vi "invatare retea.vi"() -> ()   [LabVIEW 2024]
uses:
  <vilib>/National Instruments/NI Super Simple Neural Networks/Types/Teaching Settings.ctl
  <vilib>/National Instruments/NI Super Simple Neural Networks/Types/Error Evaluation.ctl
  <vilib>/National Instruments/NI Super Simple Neural Networks/API/Create 2 Hidden Layers.vi
  <vilib>/National Instruments/NI Super Simple Neural Networks/Neural Network.lvclass
panel:
  out "F1 SCOR":dbl
  out "Accuracy":dbl
  out "Matrice confuzie":dbl[][](array[numeric])
  in  "Settings In":T1={"Max Epocs"=10000, "Error Goal"=10.0, "Max Time (s)"=10.0, "Error Evaluation"=enum."Over Teaching Set", "# Vectors per Iteration"=200}
  out "Waveform Graph 2":dbl[][](graph)
  out "Solution Found":bool
  out "Error Trend Out":dbl[](array[numeric])
  out "Teaching Time (s)":dbl
  in  "Output Layer Linear (False)":bool
  out "nume clase":string[](array[string])
  in  "2nd Hidden Layer Neurons":u32
  in  "1st Hidden Layer Neurons":u32
  # "250"
  # "60"
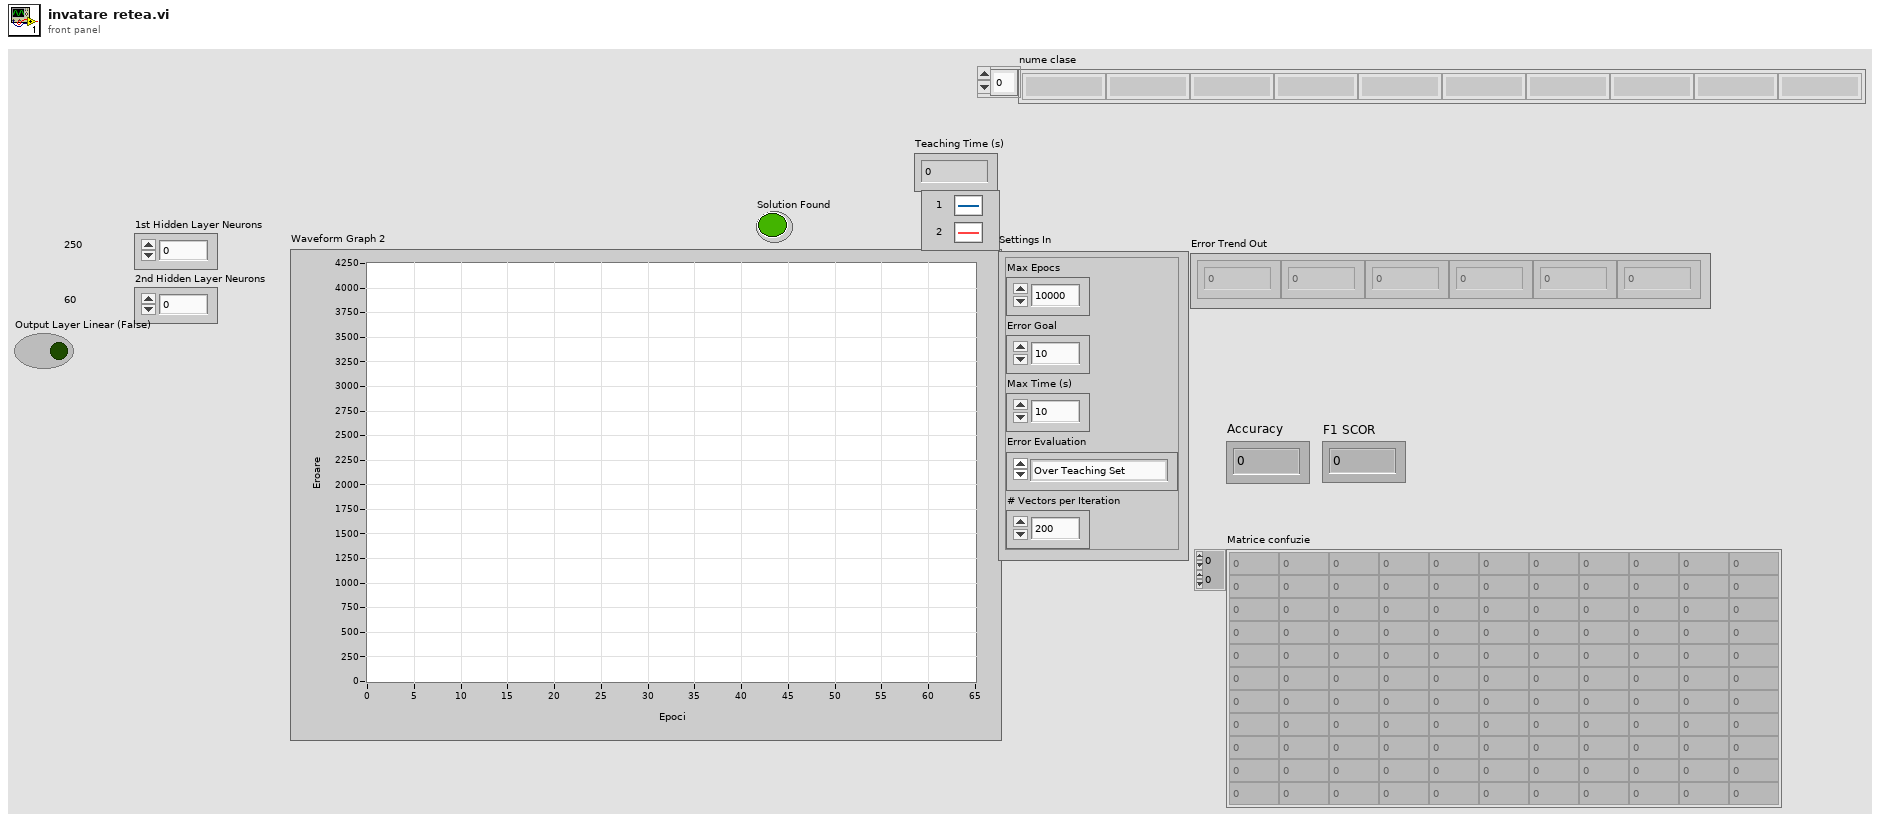
[diagram p1: front panel]
types:
  T1 = typedef "Neural Network.lvclass/Teaching Settings.ctl" = cluster{"Max Epocs":u64, "Error Goal":dbl, "Max Time (s)":dbl, "Error Evaluation":T2, "# Vectors per Iteration":i32}
  T2 = typedef "Neural Network.lvclass/Error Evaluation.ctl" = enum16{"Over Both Sets", "Over Validation Set", "Over Teaching Set"}
  T3 = typedef "imagedata.ctl" = cluster{"image type":i32, "image depth":i32, "image":u8[], "mask":u8[], "colors":u32[], "Rectangle":cluster{"left":i16, "top":i16, "right":i16, "bottom":i16}}
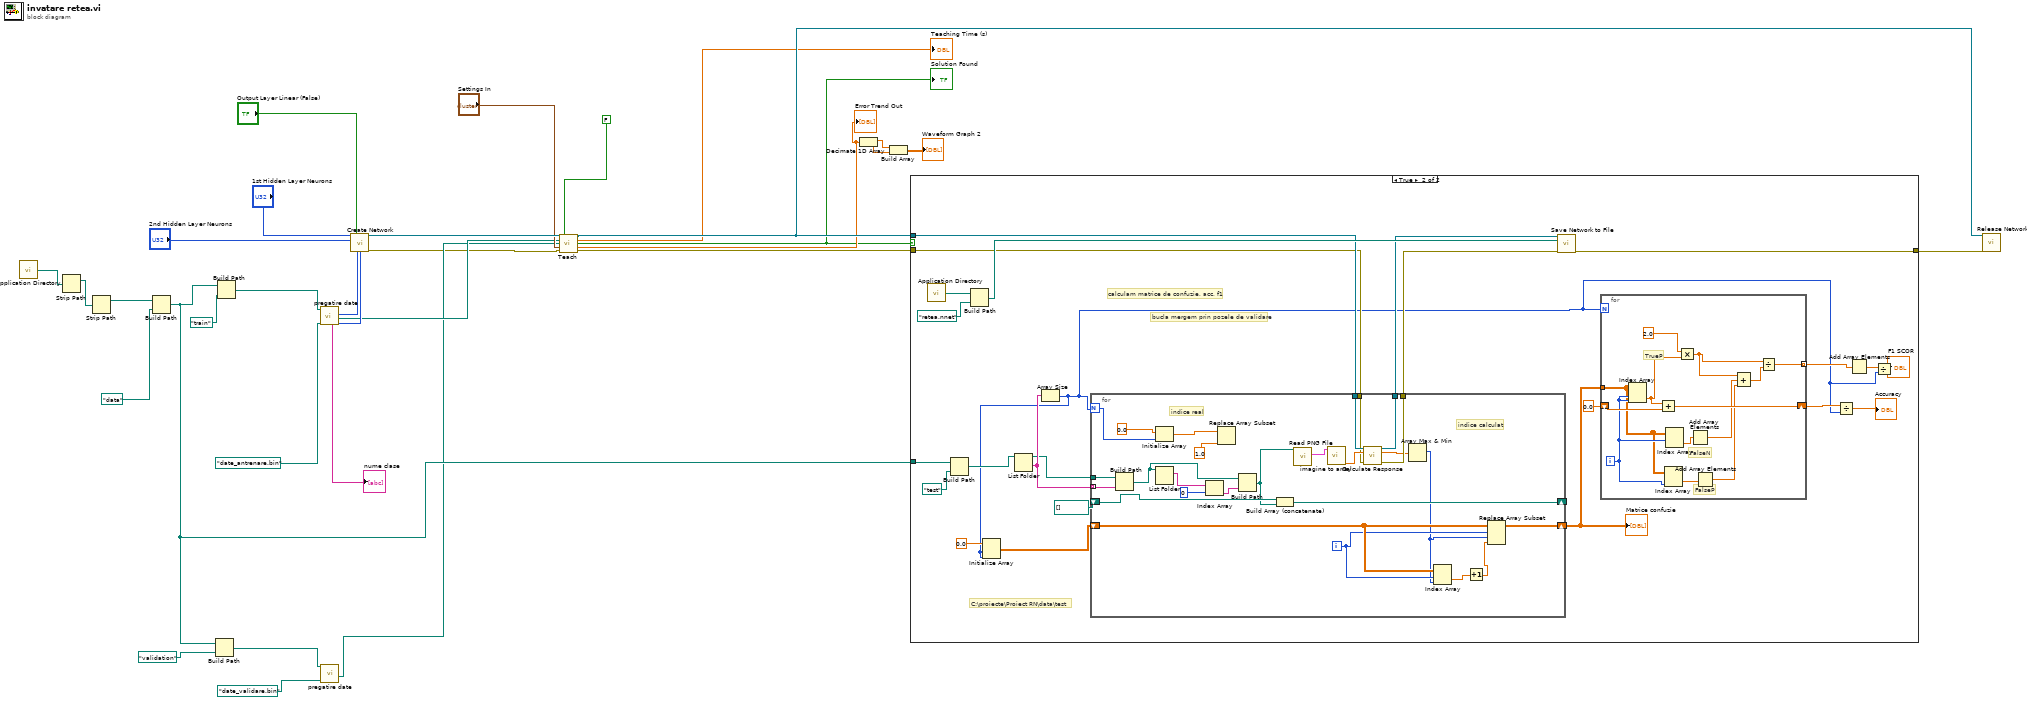
[diagram p0: block diagram]
diagram:
  n1 = call <vilib>:"Application Directory.vi"() -> ("Application Directory"=w24:path)
  n2 = Strip Path(path=w24) -> (stripped path=w23:path)  [unwired: 1 out]
  n3 = Strip Path(path=w23) -> (stripped path=w22:path)  [unwired: 1 out]
  n4 = Build Path(base path=w22, name or relative path=path "data") -> (appended path=w12:path)
  n5 = Build Path(base path=w12, name or relative path=path "validation") -> (appended path=w16:path)
  n6 = Build Path(base path=w12, name or relative path=path "train") -> (appended path=w18:path)
  n7 = call "pregatire date.vi"("nume fisier date pregatite"=path "date_antrenare.bin", "dataset folder"=w18) -> ("outputs RN"=w31:i32, "dataset trained data"=w8:path, "inputs RN"=w32:i32, "nume clase"=→"nume clase":string[])  [unwired: 5 in, 1 out]
  n8 = call "pregatire date.vi"("nume fisier date pregatite"=path "date_validare.bin", "dataset folder"=w16) -> ("dataset trained data"=w7:path)  [unwired: 5 in, 4 out]
  n9 = call-poly <vilib>:"Create Network.vi"("1st Hidden Layer Neurons"="1st Hidden Layer Neurons", "Output Layer Linear (False)"="Output Layer Linear (False)", "2nd Hidden Layer Neurons"="2nd Hidden Layer Neurons", "# Inputs"=w32, "Output Neurons/Outputs"=w31) -> ("Neural Network"=w10:refnum<class "Neural Network.lvclass">, "Error Out"=w6:errorcluster)  [unwired: 9 in]
  n10 = call <vilib>:"Teach.vi"("Neural Network In"=w10, "Enable Growing/Prunning"=FALSE, "Teaching Set Path In"=w8, "Validation Set Path In"=w7, "Settings In"="Settings In", "Error In"=w6) -> ("Neural Network Out"=w5:refnum<class "Neural Network.lvclass">, "Teaching Time (s)"=→"Teaching Time (s)":dbl, "Solution Found"=w2:bool, "Error Trend Out"=w3:dbl[], "Error Out"=w4:errorcluster)  [unwired: 5 in]
  "Error Trend Out" <- w3
  "Solution Found" <- w2
  n11 = Decimate 1D Array "Decimate 1D Array"(w3) -> (w15:dbl[], w14:dbl[])
  n12 = Build Array(w15, w14) -> (→"Waveform Graph 2":dbl[][])
  n13 = case shown="True" w2 {
    tunnel: w5 -> [_ w48]
    tunnel: w4 -> [w33 w47]
    tunnel: [w33 w57] -> w26
    tunnel: w12 -> [_ w38]
    frame False {
    }
    frame True {
      # "calculam matrice de confuzie, acc, f1"
      # "bucla mergem prin pozele de validare"
      # "C:\\proiecte\\Proiect RN\\data\\test"
      n14 = call <vilib>:"Application Directory.vi"() -> ("Application Directory"=w56:path)
      n15 = Build Path(base path=w38, name or relative path=path "test") -> (appended path=w51:path)
      n16 = Build Path(base path=w56, name or relative path=path "retea.nnet") -> (appended path=w54:path)
      n17 = List Folder(path=w51) -> (path out=w52:path, folder names=w53:string[])  [unwired: 3 in, 2 out]
      n18 = Array Size(array=w53) -> (size(s)=w35:i32)
      n19 = Initialize Array "Initialize Array"(0.0 ("element"), w35, w35) -> (w43:dbl[][])
      n20 = for {
        N: w35 -> [w79]
        tunnel: w52 -> [w96]
        shift-right: [w89] -> _
        shift-left: path[] [] -> [w95]
        tunnel: w53 -> [w94] mode=indexing
        tunnel: w48 -> [w85]
        tunnel: w47 -> [w84]
        tunnel: [w83] -> w46
        tunnel: [w82] -> w45
        shift-right: [w76] -> w42
        shift-left: w43 -> [w75]
        i -> [w72]
        # "indice real"
        # "indice calculat"
        n21 = Build Path(base path=w96, name or relative path=w94) -> (appended path=w93:path)
        n22 = Initialize Array "Initialize Array"(0.0 ("element"), w79) -> (w78:dbl[])
        n23 = List Folder(path=w93) -> (filenames=w92:string[])  [unwired: 3 in, 3 out]
        n24 = Index Array(array=w92, index=0) -> (element=w91:string)
        n25 = Replace Array Subset(array=w78, new element=1.0 ("new element/subarray")) -> ()  [unwired: 1 in, 1 out]
        n26 = Build Path(base path=w93, name or relative path=w91) -> (appended path=w88:path)
        n27 = Build Array (concatenate) "Build Array"(w95, w88) -> (w89:path[])
        n28 = call <vilib>:"Read PNG File.vi"("path to PNG file"=w88) -> ("image data"=w87:T3)  [unwired: 8 in, 2 out]
        n29 = call "imagine to array.vi"("image data"=w87) -> ("array imagine"=w86:dbl[])  [unwired: 9 in, 1 out]
        n30 = call <vilib>:"Calculate Response.vi"("Neural Network In"=w85, "Inputs"=w86, "Error In"=w84) -> ("Neural Network Out"=w83:refnum<class "Neural Network.lvclass">, "Outputs"=w81:dbl[], "Error Out"=w82:errorcluster)  [unwired: 10 in]
        n31 = Array Max & Min(array=w81) -> (max index (indices)=w71:i32)  [unwired: 3 out]
        n32 = Index Array "Index Array"(array=w75, index (row)=w72, index (col)=w71) -> (element=w74:dbl)
        n33 = Increment(x=w74) -> (x+1=w73:dbl)
        n34 = Replace Array Subset "Replace Array Subset"(array=w75, new element=w73, index (row)=w72, index (col)=w71) -> (w76:dbl[][])
      }
      "Matrice confuzie" <- w42
      n35 = call <vilib>:"Save Network to File.vi"("Neural Network In"=w46, "File Path (dialog)"=w54, "Error In"=w45) -> ("Error Out"=w57:errorcluster)  [unwired: 10 in, 2 out]
      n36 = for {
        N: w35 -> [_]
        tunnel: w42 -> [w65]
        shift-right: [w70] -> w40
        shift-left: 0.0 -> [w69]
        tunnel: [w58] -> w37 mode=indexing
        i -> [w66]
        # "FalseP"
        # "FalseN"
        # "TrueP"
        n37 = Index Array "Index Array"(array=w65, index (row)=w66, index (col)=w66) -> (element=w68:dbl)
        n38 = Add(x=w68, y=w69) -> (x+y=w70:dbl)
        n39 = Index Array "Index Array"(array=w65, index (col)=w66) -> (element=w63:dbl[])  [unwired: 1 in]
        n40 = Index Array "Index Array"(array=w65, index (row)=w66) -> (element=w64:dbl[])  [unwired: 1 in]
        n41 = Multiply(x=2.0, y=w68) -> (x*y=w62:dbl)
        n42 = Add Array Elements(numeric array=w64) -> (sum=w61:dbl)
        n43 = Add Array Elements(numeric array=w63) -> (sum=w60:dbl)
        n44 = Compound Arithmetic op=ADD(w62, w61, w60) -> (w59:dbl)
        n45 = Divide(x=w62, y=w59) -> (x/y=w58:dbl)
      }
      n46 = Divide(x=w40, y=w35) -> (x/y=→"Accuracy":dbl)
      n47 = Add Array Elements(numeric array=w37) -> (sum=w36:dbl)
      n48 = Divide(x=w36, y=w35) -> (x/y=→"F1 SCOR":dbl)
    }
  }
  n49 = call <vilib>:"Release Network.vi"("Neural Network"=w5, "Error In"=w26) -> ()  [unwired: 13 in, 1 out]
